vi "Write JSON Tree.vi"(8 "error in (no error)":errorcluster, 10 "JSON Tree":variant, 11 "params in":refnum<class "params.lvclass">) -> (0 "error out":errorcluster, 3 "params out":refnum<class "params.lvclass">)   [LabVIEW 2015]
uses:
  params.lvclass
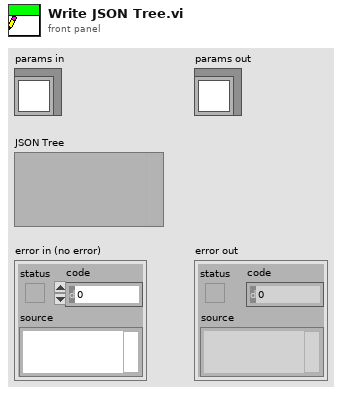
[diagram p1: front panel]
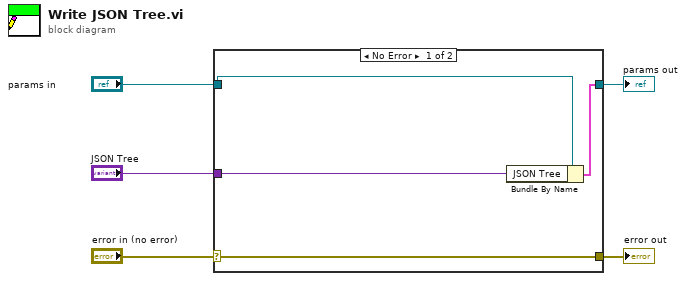
[diagram p0: block diagram]
diagram:
  n1 = case shown="No Error" "error in (no error)" {
    selector: "error in (no error)" -> [w9 w10]
    tunnel: [w9 w10] -> w4
    tunnel: [w7 w11] -> w2
    tunnel: "params in" -> [w8 w11]
    tunnel: "JSON Tree" -> [w6 _]
    frame No Error {
      n2 = Bundle By Name(cluster=w8, "JSON Tree"=w6) -> (w7:cluster{})
    }
    frame Error {
    }
  }
  "error out" <- w4
  "params out" <- w2
